vi "CODMn测量流程.vi"(11 "控制命令":u16(ring)=1 items=["启动测量"=1, "标样核查"=2, "零点核查"=3, "跨度核查"=4, "空白测试"=5, "平行样测试"=6, "加标回收"=7, "空白校准"=8, "标样校准"=9, "初始化（清洗）"=10, "停止测试"=11, "仪器重启"=12, "校时"=13, "模式设置"=14, "测量间隔设置"=15, "调试"=22, "填充管路"=30, "清洗管路"=31, "清洗反应杯"=32]) -> ()   [LabVIEW 2016, in "斯坦道CODMn新电路板.lvlib"]
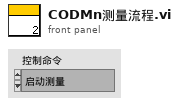
[diagram p1: front panel]
types:
  T1 = cluster{"站号":u16, "量程切换":enum32{"H", "L", "AUTO"}, "控制命令":u16, "模式设置":enum16{"待机", "连续模式", "周期模式", "定点模式", "受控模式", "手动模式"}, "测量间隔":u16}
  T2 = cluster{"系统时间":timestamp, "工作状态":u16, "测量模式":enum16{"待机", "连续模式", "周期模式", "定点模式", "受控模式", "手动模式"}, "告警代码":u16, "故障代码":u16, "日志代码":u16, "软件版本":u16, "A":sgl, "B":sgl, "K":sgl, "当前滴定数":sgl, "T":sgl, "H":sgl, "id":u16, "flowid":u16, "量程":u16, "加热实时温度":sgl, "当前ORP值":sgl, "运行时间":sgl, "当前步骤剩余时间":sgl, "结束滴定数":sgl, "注射泵保温温度":sgl, "匹配滴定数X0":u16, "X^2":sgl, "X":sgl, "B 2":sgl}
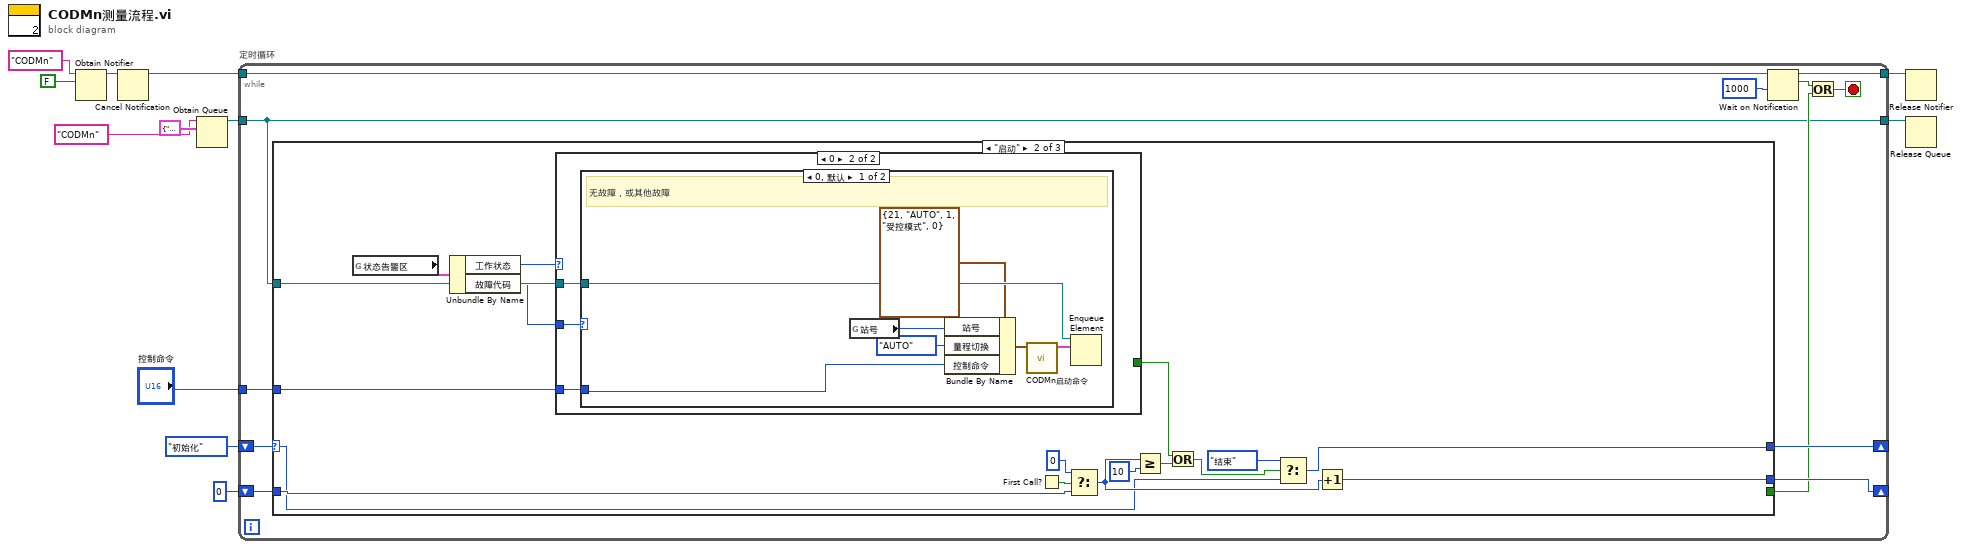
[diagram p0: block diagram]
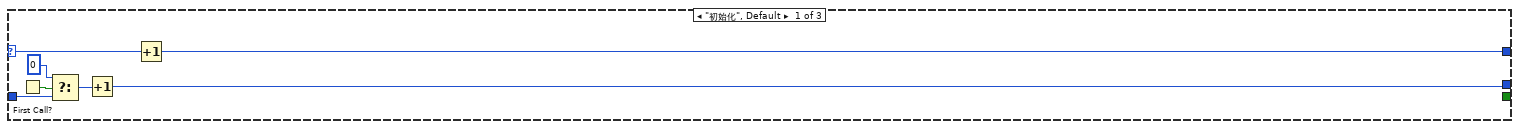
[diagram p2: hidden frame]
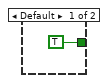
[diagram p3: hidden frame]
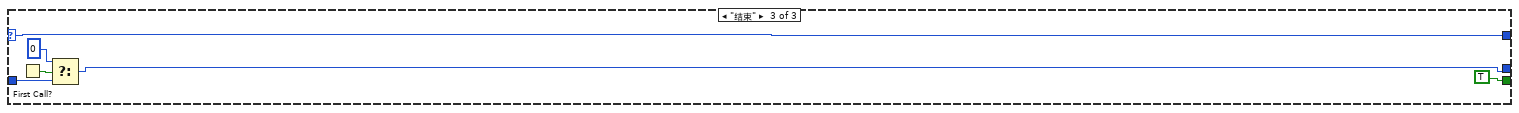
[diagram p5: hidden frame]
diagram:
  n1 = Obtain Notifier(name (unnamed)="CODMn" ("名称（未命名）"), notification data type=FALSE) -> (notifier out=w7:refnum<notifier>)  [unwired: 2 in, 2 out]
  n2 = Cancel Notification(0:w7) -> (8:w6:refnum<notifier>)  [unwired: 1 in, 2 out]
  n3 = Obtain Queue(name (unnamed)="CODMn" ("名称（未命名）"), element data type=cluster{"命令":string, "data":variant} {"命令"="", "data"=variant}) -> (queue out=w10:refnum<queue>)  [unwired: 3 in, 2 out]
  n4 = while "定时循环" {
    tunnel: w10 -> [w13]
    tunnel: w6 -> [w24]
    tunnel: "控制命令" -> [w19]
    shift-right: [w18] -> _
    shift-left: enum16{"初始化", "启动", "结束"}."初始化" -> [w20]
    shift-right: [w16] -> _
    shift-left: 0 -> [w17]
    tunnel: [w14] -> w2
    tunnel: [w13] -> w3
    stop <- w21 stop-if-true
    n5 = case shown="\"启动\"" w20 {
      selector: w20 -> [w31 w38 w65]
      tunnel: w19 -> [_ w32 _]
      tunnel: w13 -> [_ w48 _]
      tunnel: [w30 w39 w65] -> w18
      tunnel: w17 -> [w28 w43 w62]
      tunnel: [w25 w42 w61] -> w16
      tunnel: [_ _ TRUE] -> w15
      frame "初始化", Default {
        n6 = First Call?() -> (First Call?: T/F=w29:bool)
        n7 = Select(t=0, s=w29, f=w28) -> (s? t:f=w26:i32)
        n8 = Increment(x=w26) -> (x+1=w25:i32)
        n9 = Increment(x=w31) -> (x+1=w30:enum16{"初始化", "启动", "结束"})
      }
      frame "启动" {
        n10 = global read "VARCODMn全局变量.vi" "状态告警区"() -> (w47:T2)
        n11 = Unbundle By Name(w47) -> ("工作状态"=w46:u16, "故障代码"=w33:u16)
        n12 = case shown="0" w46 {
          tunnel: w32 -> [_ w51]
          tunnel: w48 -> [_ w52]
          tunnel: [TRUE _] -> w34
          tunnel: w33 -> [_ w50]
          frame Default {
          }
          frame 0 {
            n13 = case shown="0, 默认" w50 {
              tunnel: w52 -> [w58 _]
              tunnel: w51 -> [w57 _]
              frame 0, Default {
                # "无故障，或其他故障"
                n14 = global read "CODMn断电保存全局变量.vi" "站号"() -> (w56:u16)
                n15 = Bundle By Name(cluster=T1 {"站号"=21, "量程切换"=enum."AUTO", "控制命令"=1, "模式设置"=enum."受控模式", "测量间隔"=0} ("参数"), "站号"=w56, "量程切换"=enum32{"H", "L", "AUTO"}."AUTO", "控制命令"=w57) -> (w53:T1)
                n16 = call "CODMn启动命令.vi"("参数"=w53) -> ("启动命令"=w59:cluster{"命令":string, "data":variant})  [unwired: 10 in]
                n17 = Enqueue Element(queue=w58, element=w59) -> ()  [unwired: 2 in, 3 out]
              }
              frame 2 {
                # "加热故障"
              }
            }
          }
        }
        n18 = First Call?() -> (First Call?: T/F=w45:bool)
        n19 = Select(t=0, s=w45, f=w43) -> (s? t:f=w41:i32)
        n20 = Greater Or Equal?(x=w41, y=10) -> (x >= y?=w37:bool)
        n21 = Or(x=w34, y=w37) -> (x .or. y?=w35:bool)
        n22 = Select(t=enum16{"初始化", "启动", "结束"}."结束", s=w35, f=w38) -> (s? t:f=w39:enum16{"初始化", "启动", "结束"})
        n23 = Increment(x=w41) -> (x+1=w42:i32)
      }
      frame "结束" {
        n24 = First Call?() -> (First Call?: T/F=w64:bool)
        n25 = Select(t=0, s=w64, f=w62) -> (s? t:f=w61:i32)
      }
    }
    n26 = Wait on Notification(notifier=w24, timeout in ms (-1)=1000 ("超时毫秒(-1)")) -> (notifier out=w14:refnum<notifier>, notification=w22:bool)  [unwired: 2 in, 2 out]
    n27 = Or(x=w22, y=w15) -> (x .or. y?=w21:bool)
  }
  n28 = Release Notifier(notifier=w2) -> ()  [unwired: 2 in, 3 out]
  n29 = Release Queue(queue=w3) -> ()  [unwired: 2 in, 3 out]
